vi "Get Functions Type INI.vi"(8 "error in":errorcluster) -> (0 "error out":errorcluster, 3 "Function Config INI":path)   [LabVIEW 2016, in "scripts manager.lvclass"]
uses:
  scripts manager.lvclass
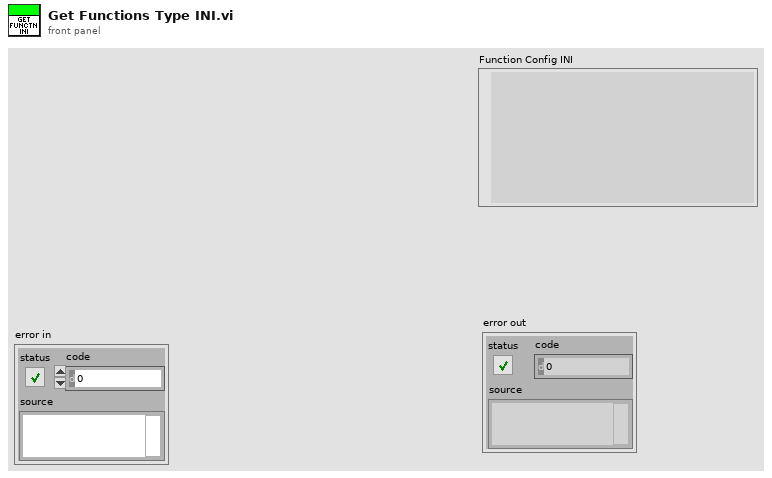
[diagram p1: front panel]
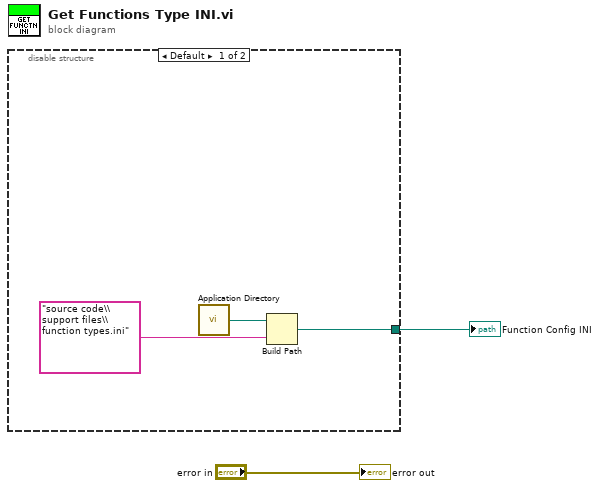
[diagram p0: block diagram]
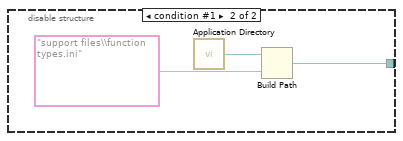
[diagram p2: hidden frame]
diagram:
  n1 = disable-structure shown="Default" {
    disable-tunnel: [w4 w7] -> w1
    frame condition #0 (active) {
      n2 = call <vilib>:"Application Directory.vi"() -> ("Application Directory"=w3:path)
      n3 = Build Path(base path=w3, name or relative path="source code\\support files\\function types.ini") -> (appended path=w4:path)
    }
    frame condition #1 {
      n4 = call <vilib>:"Application Directory.vi"() -> ("Application Directory"=w6:path)
      n5 = Build Path(base path=w6, name or relative path="support files\\function types.ini") -> (appended path=w7:path)
    }
  }
  "Function Config INI" <- w1
  "error out" <- "error in"
